vi "Archiver-RecordSequence.vi"(2 "Count":i32, 3 "file_id":i32, 7 "name":string, 9 "error in (no error)":errorcluster) -> (6 "error out":errorcluster)   [LabVIEW 2009]
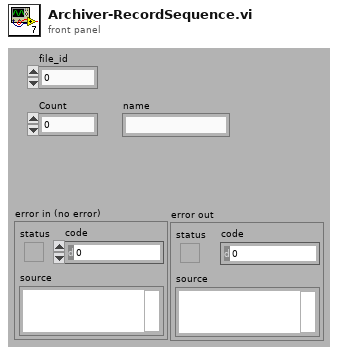
[diagram p1: front panel]
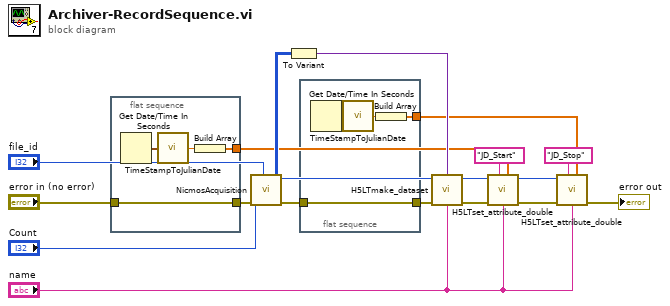
[diagram p0: block diagram]
diagram:
  n1 = flat-sequence {
    tunnel: "error in (no error)" -> [w19]
    tunnel: [w19] -> w7
    tunnel: [w17] -> w4
    frame #0 {
      n2 = Get Date/Time In Seconds() -> (seconds since 1Jan1904=w20:timestamp)
      n3 = call "TimeStampToJulianDate.vi"("TimeStamp [UT]"=w20) -> ("JulianDay"=w18:ext)
      n4 = Build Array(w18) -> (w17:ext[])
    }
  }
  n5 = call "NicmosAcquisition.vi"("Acquisition"="Count", "error in (no error)"=w7) -> ("DATA"=w10:i32[][][][], "error out"=w6:errorcluster)  [unwired: 6 in]
  n6 = To Variant(anything=w10) -> (Variant=w11:variant)
  n7 = flat-sequence {
    tunnel: w6 -> [w23]
    tunnel: [w23] -> w5
    tunnel: [w21] -> w2
    frame #0 {
      n8 = Get Date/Time In Seconds() -> (seconds since 1Jan1904=w24:timestamp)
      n9 = call "TimeStampToJulianDate.vi"("TimeStamp [UT]"=w24) -> ("JulianDay"=w22:ext)
      n10 = Build Array(w22) -> (w21:ext[])
    }
  }
  n11 = call "H5LTmake_dataset.vi"("Array"=w11, "loc_id"="file_id", "name"="name", "error in (no error)"=w5) -> ("error out"=w9:errorcluster)  [unwired: 5 in]
  n12 = call "H5LTset_attribute_double.vi"("error in (no error)"=w9, "name"="name", "loc_id"="file_id", "attr_name"="JD_Start", "buffer"=w4) -> ("error out"=w1:errorcluster)  [unwired: 5 in]
  n13 = call "H5LTset_attribute_double.vi"("error in (no error)"=w1, "name"="name", "loc_id"="file_id", "attr_name"="JD_Stop", "buffer"=w2) -> ("error out"=→"error out":errorcluster)  [unwired: 5 in]
